vi "Initialize.vi"(8 "error in (no error)":errorcluster, 11 "Time Entry-INI in":refnum<class "Time Entry-INI.lvclass">) -> (0 "error out":errorcluster, 3 "Time Entry-INI out":refnum<class "Time Entry-INI.lvclass">)   [LabVIEW 2020, in "Time Entry-INI.lvclass"]
uses:
  Time Entry-INI.lvclass
  <vilib>/Utility/sysdir.llb/System Directory Type.ctl
  Time Entry-INI.lvclass/Time Entry-INI.ctl
  Time Entry/Time Entries.lvclass
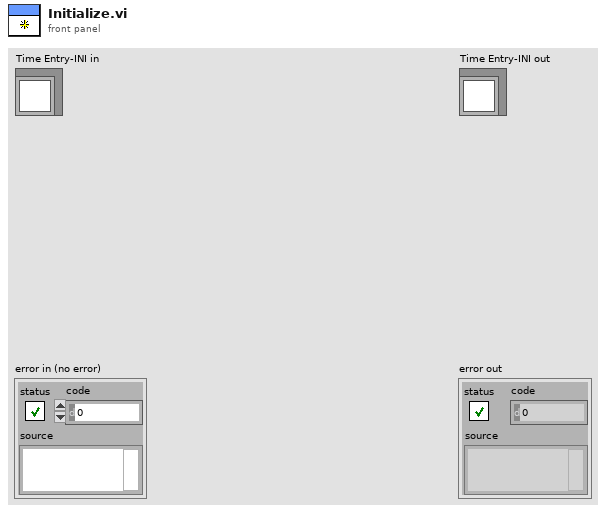
[diagram p1: front panel]
types:
  T1 = typedef "System Directory Type.ctl" = i32
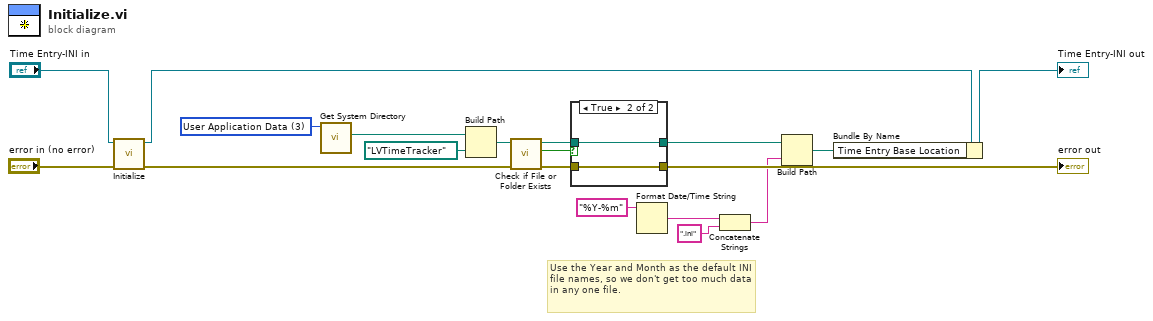
[diagram p0: block diagram]
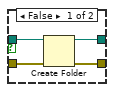
[diagram p2: hidden frame]
diagram:
  w16 = T1 3 items=["User Home"=0, "User Desktop"=1, "User Documents"=2, "User Application Data"=3, "User Preferences"=4, "User Temporary"=5, "Public Documents"=6, "Public Application Data"=7, "Public Preferences"=8, "Public Cache"=13, "System Core Libraries"=9, "System Installed Libraries"=10, "Application Files"=11, "Boot Volume Root"=12] ("system directory type")
  # "Use the Year and Month as the default INI file names, so we don't get too much data in any one file."
  n1 = call-parent "Initialize.vi"("error in (no error)"="error in (no error)", "Time Entries in"="Time Entry-INI in") -> ("error out"=w9:errorcluster, "Time Entries out"=w19:refnum<class "Time Entry-INI.lvclass">)  [unwired: 8 in]
  n2 = call <vilib>:"Get System Directory.vi"("system directory type"=w16) -> ("system directory"=w15:path)  [unwired: 10 in]
  n3 = Build Path(base path=w15, name or relative path=path "LVTimeTracker") -> (appended path=w13:path)
  n4 = call <vilib>:"Check if File or Folder Exists.vi"("error in (no error)"=w9, "path"=w13) -> ("error out"=w10:errorcluster, "file or folder exists?"=w12:bool, "dup path"=w11:path)  [unwired: 7 in]
  n5 = case shown="True" w12 {
    tunnel: w11 -> [w23 w25]
    tunnel: w10 -> [w22 w24]
    tunnel: [w21 w24] -> w7
    tunnel: [w20 w25] -> w3
    frame False {
      n6 = Create Folder(path (use dialog)=w23, error in=w22) -> (created path=w20:path, error out=w21:errorcluster)  [unwired: 1 in, 1 out]
    }
    frame True {
    }
  }
  "error out" <- w7
  n7 = Format Date/Time String(time format string (%c)="%Y-%m") -> (date/time string=w5:string)  [unwired: 2 in]
  n8 = Concatenate Strings(w5, ".ini" ("time format string (%c)")) -> (w2:string)
  n9 = Build Path(base path=w3, name or relative path=w2) -> (appended path=w1:path)
  n10 = Bundle By Name(cluster=w19, "Time Entry Base Location"=w1) -> (→"Time Entry-INI out":refnum<class "Time Entry-INI.lvclass">)
